vi "Sys config window-Exit dialogue.vi"(11 "Initial Configuration":T2={"Triggers output setup"=[], "General trigger settings"={"Trigger 1 function"=enum."Line trigger", "Triggers loop clock (MHz)"=115.0}, "Calibration settings"={"Pockels cal.Zoom"=0, "Pockels cal.Dwell time (µs)"=0.0}, "Hardware Configuration"={"Dev. PC"=FALSE, "Swap XY on stage"=FALSE, "No of AOD"=0, "Computer MAC address"="", "Externalise Triggers"=FALSE, "Trigger HW config"={"Available Device List"=0, "Device Address"=""}, "DAQmx Chan"={"Pockels AO"="", "Hard shutter AO"="", "PMT AOs"="", "Galvo AOs"="", "Power meter AI"=""}, "XY stage available"=FALSE, "XY Stage"={"COM port"="", "Baudrate"=0, "Type"=""}, "Z stage available"=FALSE, "Z Stage config cluster"={"COM port"="COM7", "Baudrate"=0, "Type"=""}, "Encoder available"=FALSE, "Encoder"={"IP address"="224.0.1.103", "Port"=7000, "Wheel radius (cm)"=16.0, "Encoder Trigger"=""}, "VidRec available"=FALSE, "Cam VidRec"={"DO flag-Video record"="", "DO flag-Trial start"=""}, "Laser Power Control HW config"={"Laser Power Control"="", "Laser Power Modulation Control"=enum."NI"}, "Laser 1 available"=FALSE, "Laser 1 config cluster"={"COM port"="COM7", "Baud Rate"=0, "Type"=""}, "Prechirper 1 available"=FALSE, "Prechirper 1 config cluster"={"Type"="", "Baud Rate"=0, "COM port"="COM7"}, "Control system.FPGA available?"=FALSE, "Control Sys. HW config"={"Control system.FPGA Type"=enum."Virtex 5", "Control system.Network adapter name"="", "Control system.MAC address"="", "Control system.Ethernet Port"=0, "Control system.Ethernet Port Opened"=FALSE}, "DAQ FPGA HW Config"={"FGPA Ref"=refnum, "Target"="RIO0", "input card type"=enum."AC Card"}}, "System Config"={"Laser wavelength (nm)"=920.0, "DAQ FPGA System"={"Clock Freq (MHz) "=200.0, "Samples Wait after Trigger"=5080, "AOD fill"=4900, "StartupDelay"=0, "Slip Cycle (clock cycles)"=600000, "Add Cycle"=TRUE}, "Control system"={"AOD 1 Amplitude"=0, "AOD 2 Amplitude"=0, "AOD 3 Amplitude"=0, "AOD 4 Amplitude"=0, "AOD 5 Amplitude"=0, "AOD 6 Amplitude"=0, "T0 (ns)"=0.0, "Ta (ns)"=0.0, "Data Time Interval (ns)"=0.0, "Ctrl FPGA Clock (MHz)"=240.0}}, "Calibration config."={"Current Objective"="", "Objective Settings"=[], "PreChirper Values Preset ?"=FALSE, "PreChirper Settings"=[], "PreChirper Constants"={"a 1"=0, "b 1"=0, "c 1"=0, "a 2"=0, "b 2"=0, "c 2"=0, "lmin"=0, "lmax"=0}}, "General Setup"={"Microscope ID"="003", "Microscope Type"="AOLM", "Revision Number"="1.0.0.0", "Advanced Imaging"=FALSE, "Error Logging"=FALSE, "Performance Monitoring"=FALSE, "Max Allowed Trial Length"=60.0, "Initial Scan Resolution"=512.0, "Initial Acceptance Angle"=5.0, "Initial Laser Wavelength"=900.0, "Initial Dwell Time"=900.0}, "AOD Settings - distilled"={"AOD 1 thickness (mm)"=0.0, "AOD 2 thickness (mm)"=0.0, "AOD 3 thickness (mm)"=110.0, "AOD 4 thickness (mm)"=135.0, "AOD 1-2 separation (mm)"=15.0, "AOD 2-3 separation (mm)"=15.0, "AOD 3-4 separation (mm)"=15.0, "AOD 1 Centre (mm)"=15.0, "AOD 2 Centre (mm)"=50.0, "AOD 3 Centre (mm)"=50.0, "AOD 4 Centre (mm)"=50.0, "AOD 1 X Offset"=15.0, "AOD 2 X Offset"=1.0, "AOD 3 X Offset"=1.0, "AOD 4 X Offset"=1.0, "AOD 1 Y Offset"=1.0, "AOD 2 Y Offset"=1.0, "AOD 3 Y Offset"=1.0, "AOD 4 Y Offset"=1.0, "Timing Offset AOD 1"=0.0, "Timing Offset AOD 2"=0.0, "Timing Offset AOD 3"=0.0, "Timing Offset AOD 4"=0.0, "AOL centre wavelength (nm)"=1.0, "AOL centre frequency (MHz)"=1.0, "Pair deflection ratio"=1.0, "AOL aperture (mm)"=0.0, "AOD fill time (us)"=0.0, "Diffraction mode"=0.0, "Crystal length (mm)"=0.0, "Acoustic velocity (m/s)"=1.0, "AOD Ord. Refractive index"=20000.0}} {"System Config"."Control system"."Ctrl FPGA Clock (MHz)" min=80.0 max=500.0 step=1.0; "System Config"."Control system"."Data Time Interval (ns)" min=0.0 max=2048.0 step=1.0; "System Config"."Control system"."Ta (ns)" min=0.0 max=2048.0 step=1.0; "System Config"."Control system"."T0 (ns)" min=0.0 max=2048.0 step=1.0; "System Config"."Control system"."AOD 6 Amplitude" min=0 max=2048 step=1; "System Config"."Control system"."AOD 5 Amplitude" min=0 max=2048 step=1; "System Config"."Control system"."AOD 4 Amplitude" min=0 max=2048 step=1; "System Config"."Control system"."AOD 3 Amplitude" min=0 max=2048 step=1; "System Config"."Control system"."AOD 2 Amplitude" min=0 max=2048 step=1; "System Config"."Control system"."AOD 1 Amplitude" min=0 max=2048 step=1; "System Config"."Laser wavelength (nm)" min=800.0 max=1080.0 step=1.0; "Hardware Configuration"."Encoder"."Wheel radius (cm)" format="%#_13g"; "General trigger settings"."Triggers loop clock (MHz)" format="%#_13g"; "Triggers output setup"."Pulse width (us)" min=10 max=5000 step=1 format="%.0fµs"}) -> (3 "Close":bool)   [LabVIEW 2017]
uses:
  Configuration code/Typedefs/Initial config.ctl
  Peripherals Control/Triggers/Typedefs/Triggers output setup.ctl
  Peripherals Control/Triggers/Typedefs/Trigger setup element cluster.ctl
  Peripherals Control/Triggers/Typedefs/General trigger settings cluster.ctl
  Typedefs/Trigger 1 selector enum.ctl
  Configuration code/Typedefs/Pockels Calibration settings cluster.ctl
  Typedefs/Hardware Configuration settings.ctl
  Typedefs/Triggers HW config.ctl
  Typedefs/DAQmx physical channels cluster.ctl
  Typedefs/XY Stage config cluster.ctl
  Typedefs/Z Stage config cluster.ctl
  Typedefs/Encoder config cluster.ctl
  Typedefs/Cam VidRec HW config setup cluster.ctl
  Typedefs/Laser Power Control HW config.ctl
  Typedefs/Laser 1 config cluster.ctl
  Typedefs/PreChirper 1 config cluster.ctl
  Typedefs/Control Sys HW config cluster.ctl
  Typedefs/DAQ FPGA HW config cluster.ctl
  RIG-SPECIFIC FILES/FPGA Refs/FPGA Ref.ctl
  <vilib>/userdefined/High Color/nirio_resource_hc.ctl
  Typedefs/FPGA input type AC-DC.ctl
  Typedefs/System Configuration.ctl
  Typedefs/DAQ FPGA system config.ctl
  Typedefs/CTRL system config.ctl
  Typedefs/Calibration config.ctl
  Typedefs/Objective Config.ctl
  Typedefs/Prechirper Cal Config.ctl
  Typedefs/PreChirper constants.ctl
  Typedefs/General Setup.ctl
  Typedefs/AOD Settings-distilled.ctl
  Visualisation/Functional Imaging Viewer/Typedefs/Get-Set-Clear Control.ctl
panel:
  out "x != y?":T1
  # "Thickness (mm)"
  # "X Offset"
  # "Separation (mm)"
  # "Y Offset"
  # "Centre (mm)"
  # "Timing Offset"
types:
  T1 = cluster{"Triggers output setup":cluster{"Name":bool, "Output?":bool, "Output terminal":bool, "PXI backplane line":bool, "Pulse width (us)":bool}[], "General trigger settings":cluster{"Trigger 1 function":bool, "Triggers loop clock (MHz)":bool}, "Calibration settings":cluster{"Pockels cal.Zoom":bool, "Pockels cal.Dwell time (µs)":bool}, "Hardware Configuration":cluster{"Dev. PC":bool, "Swap XY on stage":bool, "No of AOD":bool, "Computer MAC address":bool, "Externalise Triggers":bool, "Trigger HW config":cluster{"Available Device List":bool, "Device Address":bool}, "DAQmx Chan":cluster{"Pockels AO":bool, "Hard shutter AO":bool, "PMT AOs":bool, "Galvo AOs":bool, "Power meter AI":bool}, "XY stage available":bool, "XY Stage":cluster{"COM port":bool, "Baudrate":bool, "Type":bool}, "Z stage available":bool, "Z Stage config cluster":cluster{"COM port":bool, "Baudrate":bool, "Type":bool}, "Encoder available":bool, "Encoder":cluster{"IP address":bool, "Port":bool, "Wheel radius (cm)":bool, "Encoder Trigger":bool}, "VidRec available":bool, "Cam VidRec":cluster{"DO flag-Video record":bool, "DO flag-Trial start":bool}, "Laser Power Control HW config":cluster{"Laser Power Control":bool, "Laser Power Modulation Control":bool}, "Laser 1 available":bool, "Laser 1 config cluster":cluster{"COM port":bool, "Baud Rate":bool, "Type":bool}, "Prechirper 1 available":bool, "Prechirper 1 config cluster":cluster{"Type":bool, "Baud Rate":bool, "COM port":bool}, "Control system.FPGA available?":bool, "Control Sys. HW config":cluster{"Control system.FPGA Type":bool, "Control system.Network adapter name":bool, "Control system.MAC address":bool, "Control system.Ethernet Port":bool, "Control system.Ethernet Port Opened":bool}, "DAQ FPGA HW Config":cluster{"FGPA Ref":bool, "Target":bool, "input card type":bool}}, "System Config":cluster{"Laser wavelength (nm)":bool, "DAQ FPGA System":cluster{"Clock Freq (MHz) ":bool, "Samples Wait after Trigger":bool, "AOD fill":bool, "StartupDelay":bool, "Slip Cycle (clock cycles)":bool, "Add Cycle":bool}, "Control system":cluster{"AOD 1 Amplitude":bool, "AOD 2 Amplitude":bool, "AOD 3 Amplitude":bool, "AOD 4 Amplitude":bool, "AOD 5 Amplitude":bool, "AOD 6 Amplitude":bool, "T0 (ns)":bool, "Ta (ns)":bool, "Data Time Interval (ns)":bool, "Ctrl FPGA Clock (MHz)":bool}}, "Calibration config.":cluster{"Current Objective":bool, "Objective Settings":cluster{"Name":bool, "Sum X":bool, "Sum Y":bool, "Diff X":bool, "Diff Y":bool, "Distortion Correction":bool, "Z_norm to um_scaling":bool, "X_norm to um_scaling":bool, "Calibrated Wavelength":bool}[], "PreChirper Values Preset ?":bool, "PreChirper Settings":cluster{"Wavelength":bool, "Prism 1":bool, "Prism 2":bool}[], "PreChirper Constants":cluster{"a 1":bool, "b 1":bool, "c 1":bool, "a 2":bool, "b 2":bool, "c 2":bool, "lmin":bool, "lmax":bool}}, "General Setup":cluster{"Microscope ID":bool, "Microscope Type":bool, "Revision Number":bool, "Advanced Imaging":bool, "Error Logging":bool, "Performance Monitoring":bool, "Max Allowed Trial Length":bool, "Initial Scan Resolution":bool, "Initial Acceptance Angle":bool, "Initial Laser Wavelength":bool, "Initial Dwell Time":bool}, "AOD Settings - distilled":cluster{"AOD 1 thickness (mm)":bool, "AOD 2 thickness (mm)":bool, "AOD 3 thickness (mm)":bool, "AOD 4 thickness (mm)":bool, "AOD 1-2 separation (mm)":bool, "AOD 2-3 separation (mm)":bool, "AOD 3-4 separation (mm)":bool, "AOD 1 Centre (mm)":bool, "AOD 2 Centre (mm)":bool, "AOD 3 Centre (mm)":bool, "AOD 4 Centre (mm)":bool, "AOD 1 X Offset":bool, "AOD 2 X Offset":bool, "AOD 3 X Offset":bool, "AOD 4 X Offset":bool, "AOD 1 Y Offset":bool, "AOD 2 Y Offset":bool, "AOD 3 Y Offset":bool, "AOD 4 Y Offset":bool, "Timing Offset AOD 1":bool, "Timing Offset AOD 2":bool, "Timing Offset AOD 3":bool, "Timing Offset AOD 4":bool, "AOL centre wavelength (nm)":bool, "AOL centre frequency (MHz)":bool, "Pair deflection ratio":bool, "AOL aperture (mm)":bool, "AOD fill time (us)":bool, "Diffraction mode":bool, "Crystal length (mm)":bool, "Acoustic velocity (m/s)":bool, "AOD Ord. Refractive index":bool}}
  T2 = typedef "Initial config.ctl" = cluster{"Triggers output setup":T3, "General trigger settings":T5, "Calibration settings":T7, "Hardware Configuration":T8, "System Config":T23, "Calibration config.":T26, "General Setup":T30, "AOD Settings - distilled":T31}
  T3 = typedef "Triggers output setup.ctl" = T4[]
  T4 = typedef "Trigger setup element cluster.ctl" = cluster{"Name":string, "Output?":bool, "Output terminal":tag, "PXI backplane line":tag, "Pulse width (us)":u16}
  T5 = typedef "General trigger settings cluster.ctl" = cluster{"Trigger 1 function":T6, "Triggers loop clock (MHz)":dbl}
  T6 = typedef "Trigger 1 selector enum.ctl" = enum16{"Encoder trigger", "Line trigger", "Control system's ref frame acknowledgement"}
  T7 = typedef "Pockels Calibration settings cluster.ctl" = cluster{"Pockels cal.Zoom":u8, "Pockels cal.Dwell time (µs)":dbl}
  T8 = typedef "Hardware Configuration settings.ctl" = cluster{"Dev. PC":bool, "Swap XY on stage":bool, "No of AOD":u8, "Computer MAC address":string, "Externalise Triggers":bool, "Trigger HW config":T9, "DAQmx Chan":T10, "XY stage available":bool, "XY Stage":T11, "Z stage available":bool, "Z Stage config cluster":T12, "Encoder available":bool, "Encoder":T13, "VidRec available":bool, "Cam VidRec":T14, "Laser Power Control HW config":T15, "Laser 1 available":bool, "Laser 1 config cluster":T16, "Prechirper 1 available":bool, "Prechirper 1 config cluster":T17, "Control system.FPGA available?":bool, "Control Sys. HW config":T18, "DAQ FPGA HW Config":T19}
  T9 = typedef "Triggers HW config.ctl" = cluster{"Available Device List":i32, "Device Address":string}
  T10 = typedef "DAQmx physical channels cluster.ctl" = cluster{"Pockels AO":tag, "Hard shutter AO":tag, "PMT AOs":tag, "Galvo AOs":tag, "Power meter AI":tag}
  T11 = typedef "XY Stage config cluster.ctl" = cluster{"COM port":refnum<visa-resource-name>, "Baudrate":i32, "Type":string}
  T12 = typedef "Z Stage config cluster.ctl" = cluster{"COM port":refnum<visa-resource-name>, "Baudrate":i32, "Type":string}
  T13 = typedef "Encoder config cluster.ctl" = cluster{"IP address":string, "Port":u16, "Wheel radius (cm)":dbl, "Encoder Trigger":tag}
  T14 = typedef "Cam VidRec HW config setup cluster.ctl" = cluster{"DO flag-Video record":tag, "DO flag-Trial start":tag}
  T15 = typedef "Laser Power Control HW config.ctl" = cluster{"Laser Power Control":string, "Laser Power Modulation Control":enum16{"NI", "FPGA"}}
  T16 = typedef "Laser 1 config cluster.ctl" = cluster{"COM port":refnum<visa-resource-name>, "Baud Rate":i32, "Type":string}
  T17 = typedef "PreChirper 1 config cluster.ctl" = cluster{"Type":string, "Baud Rate":i32, "COM port":refnum<visa-resource-name>}
  T18 = typedef "Control Sys HW config cluster.ctl" = cluster{"Control system.FPGA Type":enum16{"Virtex 5", "Virtex 7"}, "Control system.Network adapter name":string, "Control system.MAC address":string, "Control system.Ethernet Port":u32, "Control system.Ethernet Port Opened":bool}
  T19 = typedef "DAQ FPGA HW config cluster.ctl" = cluster{"FGPA Ref":T20, "Target":T21, "input card type":T22}
  T20 = typedef "FPGA Ref.ctl" = refnum<k20>
  T21 = typedef "nirio_resource_hc.ctl" = tag
  T22 = typedef "FPGA input type AC-DC.ctl" = enum16{"AC Card", "DC Card"}
  T23 = typedef "System Configuration.ctl" = cluster{"Laser wavelength (nm)":dbl, "DAQ FPGA System":T24, "Control system":T25}
  T24 = typedef "DAQ FPGA system config.ctl" = cluster{"Clock Freq (MHz) ":dbl, "Samples Wait after Trigger":u16, "AOD fill":u16, "StartupDelay":i32, "Slip Cycle (clock cycles)":u32, "Add Cycle":bool}
  T25 = typedef "CTRL system config.ctl" = cluster{"AOD 1 Amplitude":i16, "AOD 2 Amplitude":i16, "AOD 3 Amplitude":i16, "AOD 4 Amplitude":i16, "AOD 5 Amplitude":i16, "AOD 6 Amplitude":i16, "T0 (ns)":dbl, "Ta (ns)":dbl, "Data Time Interval (ns)":dbl, "Ctrl FPGA Clock (MHz)":dbl}
  T26 = typedef "Calibration config.ctl" = cluster{"Current Objective":string, "Objective Settings":T27[], "PreChirper Values Preset ?":bool, "PreChirper Settings":T28[], "PreChirper Constants":T29}
  T27 = typedef "Objective Config.ctl" = cluster{"Name":string, "Sum X":dbl, "Sum Y":dbl, "Diff X":dbl, "Diff Y":dbl, "Distortion Correction":dbl, "Z_norm to um_scaling":dbl, "X_norm to um_scaling":dbl, "Calibrated Wavelength":dbl}
  T28 = typedef "Prechirper Cal Config.ctl" = cluster{"Wavelength":i32, "Prism 1":i32, "Prism 2":i32}
  T29 = typedef "PreChirper constants.ctl" = cluster{"a 1":i32, "b 1":i32, "c 1":i32, "a 2":i32, "b 2":i32, "c 2":i32, "lmin":i32, "lmax":i32}
  T30 = typedef "General Setup.ctl" = cluster{"Microscope ID":string, "Microscope Type":string, "Revision Number":string, "Advanced Imaging":bool, "Error Logging":bool, "Performance Monitoring":bool, "Max Allowed Trial Length":dbl, "Initial Scan Resolution":dbl, "Initial Acceptance Angle":dbl, "Initial Laser Wavelength":dbl, "Initial Dwell Time":dbl}
  T31 = typedef "AOD Settings-distilled.ctl" = cluster{"AOD 1 thickness (mm)":dbl, "AOD 2 thickness (mm)":dbl, "AOD 3 thickness (mm)":dbl, "AOD 4 thickness (mm)":dbl, "AOD 1-2 separation (mm)":dbl, "AOD 2-3 separation (mm)":dbl, "AOD 3-4 separation (mm)":dbl, "AOD 1 Centre (mm)":dbl, "AOD 2 Centre (mm)":dbl, "AOD 3 Centre (mm)":dbl, "AOD 4 Centre (mm)":dbl, "AOD 1 X Offset":dbl, "AOD 2 X Offset":dbl, "AOD 3 X Offset":dbl, "AOD 4 X Offset":dbl, "AOD 1 Y Offset":dbl, "AOD 2 Y Offset":dbl, "AOD 3 Y Offset":dbl, "AOD 4 Y Offset":dbl, "Timing Offset AOD 1":dbl, "Timing Offset AOD 2":dbl, "Timing Offset AOD 3":dbl, "Timing Offset AOD 4":dbl, "AOL centre wavelength (nm)":dbl, "AOL centre frequency (MHz)":dbl, "Pair deflection ratio":dbl, "AOL aperture (mm)":dbl, "AOD fill time (us)":dbl, "Diffraction mode":dbl, "Crystal length (mm)":dbl, "Acoustic velocity (m/s)":dbl, "AOD Ord. Refractive index":dbl}
  T32 = typedef "Get-Set-Clear Control.ctl" = enum16{"Get", "Set", "Clear"}
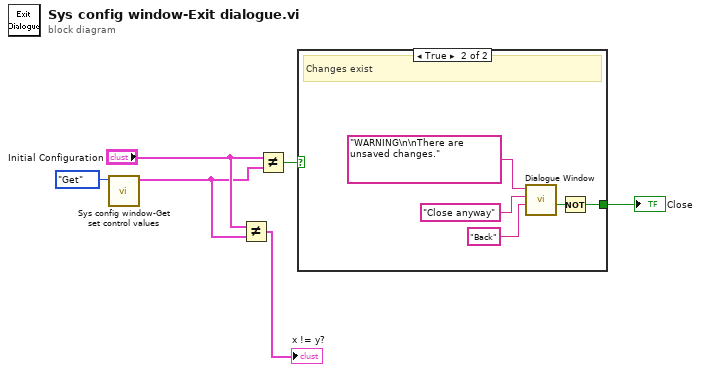
[diagram p0: block diagram]
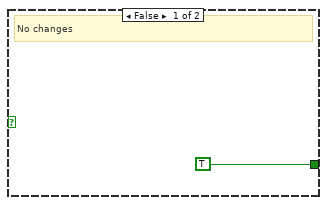
[diagram p2: hidden frame]
diagram:
  n1 = call "Sys config window-Get set control values.vi"("Function"=Get-Set-Clear_Control."Get") -> ("output cluster"=w2:T2)  [unwired: 9 in, 1 out]
  n2 = Not Equal?(x="Initial Configuration", y=w2) -> (x != y?=→"x != y?":T1)
  n3 = Not Equal?(x="Initial Configuration", y=w2) -> (x != y?=w5:bool)
  n4 = case shown="True" w5 {
    tunnel: [TRUE ("Close") w8] -> w6
    frame False {
      # "No changes"
    }
    frame True {
      # "Changes exist"
      n5 = call "Dialogue Window.vi"("Caption-Left button (Cancel)"="Back" ("Caption-Right button (OK)"), "Caption-Right button (OK)"="Close anyway" ("Caption-Left button (Cancel)"), "Message string"="WARNING\n\nThere are unsaved changes.") -> ("Cancelled (Left button pressed)"=w9:bool)  [unwired: 6 in, 2 out]
      n6 = Not(x=w9) -> (.not. x?=w8:bool)
    }
  }
  "Close" <- w6
